vi "LaunchControlPanel.vi"() -> ()   [LabVIEW 2014, in "zsLaunch.lvlib" / "Launcher.lvclass"]
uses:
  Launcher.lvclass
  ctl/P3AT_Ini.ctl
  <vilib>/Utility/xml.llb/Write to XML File.vi
  <vilib>/ActorFramework/Actor/Actor.lvclass
  ControlPanel_lib/Input Operator/ControlPanel.lvclass
panel:
  out "XML String":string caption="XML字符串"
  in  "P3AT_Ini":T1={"Is_Dirty"=FALSE, "max_vel"=0.18867924528301885, "max_rot"=0.16981132075471697, "Ini_pose_X"=0.0, "Ini_pose_Y"=0.0, "Ini_pose_Rot_deg"=0.0, "Control_Mode"=enum."Joy", "布尔"=FALSE} {"max_rot" scale=0.0..1.0; "max_vel" scale=0.0..1.0}
  out "error out":errorcluster caption="错误输出"
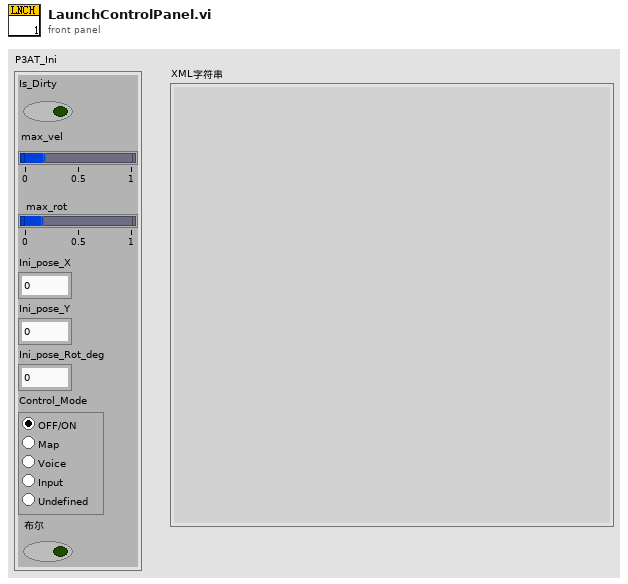
[diagram p1: front panel]
types:
  T1 = typedef "P3AT_Ini.ctl" = cluster{"Is_Dirty":bool, "max_vel":dbl, "max_rot":dbl, "Ini_pose_X":dbl, "Ini_pose_Y":dbl, "Ini_pose_Rot_deg":dbl, "Control_Mode":enum32{"Joy", "Map", "Voice", "Input", "Undefined"}, "布尔":bool}
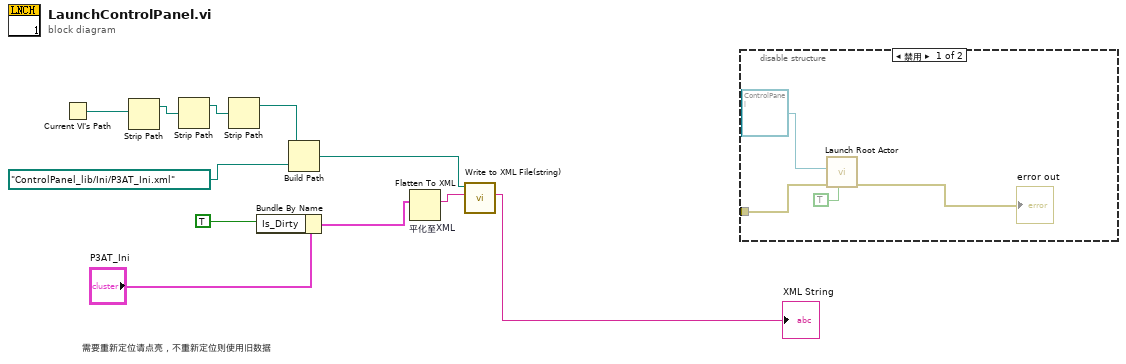
[diagram p0: block diagram]
diagram:
  # "需要重新定位请点亮，不重新定位则使用旧数据"
  n1 = Current VI's Path() -> (path=w10:path)
  n2 = Strip Path(path=w10) -> (stripped path=w9:path)  [unwired: 1 out]
  n3 = Strip Path(path=w9) -> (stripped path=w8:path)  [unwired: 1 out]
  n4 = Strip Path(path=w8) -> (stripped path=w7:path)  [unwired: 1 out]
  n5 = Bundle By Name(cluster="P3AT_Ini", "Is_Dirty"=TRUE ("重新定位？")) -> (w1:T1)
  n6 = Build Path(base path=w7, name or relative path=path "ControlPanel_lib/Ini/P3AT_Ini.xml" ("拆分的路径")) -> (appended path=w5:path)
  n7 = Flatten To XML "平化至XML"(anything=w1) -> (xml string=w11:string)
  n8 = call-poly <vilib>:"Write to XML File(string).vi"("XML Input"=w11, "XML File Path"=w5) -> ("XML String"=→"XML String":string)  [unwired: 3 in, 6 out]
  n9 = disable-structure shown="禁用" {
    disable-tunnel: _ -> [w12 _]
    frame Disabled {
      n10 = call <vilib>:"Launch Root Actor.vi"("Open Actor Core front panel? (F)"=TRUE, "error in (no error)"=w12, "Actor"=refnum<class "ControlPanel.lvclass"> refnum ("ControlPanel.lvlib:ControlPanel.lvclass")) -> ("error out"=→"error out":errorcluster)  [unwired: 7 in, 1 out]
    }
    frame Enabled {
    }
  }
